vi "Read K_ff.vi"(8 "error in (no error)":errorcluster, 11 "Altitude Guidance in":refnum<class "Altitude Guidance.lvclass">) -> (0 "error out":errorcluster, 2 "K_ff":dbl, 3 "Altitude Guidance out":refnum<class "Altitude Guidance.lvclass">)   [LabVIEW 2014, in "Guidance Library.lvlib" / "Altitude Guidance.lvclass"]
uses:
  Altitude Guidance.lvclass
  Altitude Guidance.lvclass/Altitude Guidance.ctl
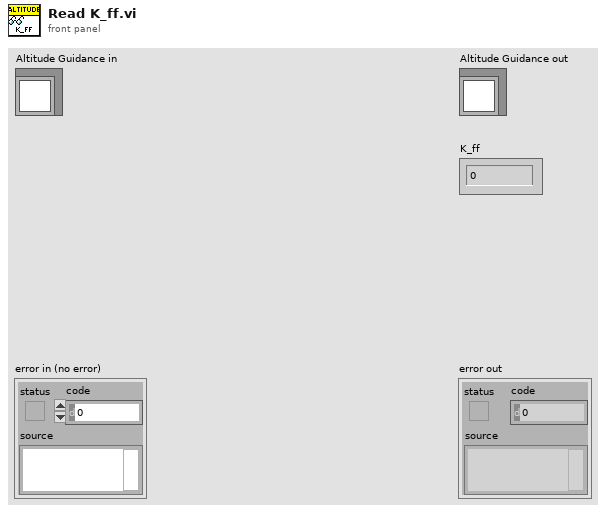
[diagram p1: front panel]
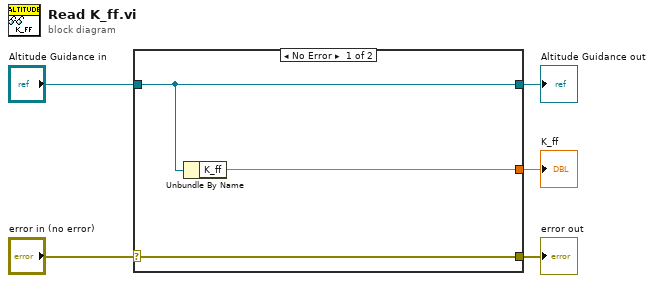
[diagram p0: block diagram]
diagram:
  n1 = case shown="No Error" "error in (no error)" {
    selector: "error in (no error)" -> [w8 w9]
    tunnel: [w8 w9] -> w4
    tunnel: [w7 w10] -> w2
    tunnel: "Altitude Guidance in" -> [w7 w10]
    tunnel: [w6 _] -> w1
    frame No Error {
      n2 = Unbundle By Name(w7) -> ("K_ff"=w6:dbl)
    }
    frame Error {
    }
  }
  "error out" <- w4
  "Altitude Guidance out" <- w2
  "K_ff" <- w1
